vi "SVFA Power Spectral Density Subset (N Ch).vi"(0 "scaled signals [EU]":waveform(dbl)[](array[waveform]), 2 "window":T7=1 items=["None"=0, "Hanning"=1, "Hamming"=2, "Blackman-Harris"=3, "Exact Blackman"=4, "Blackman"=5, "Flat Top"=6, "4 Term B-Harris "=7, "7 Term B-Harris"=8, "Low Sidelobe"=9, "Force"=64, "Exponential"=65, "Blackman Nuttall"=11, "Triangle"=30, "Bartlett-Hanning"=31, "Bohman"=32, "Parzen"=33, "Welch"=34, "Kaiser"=60, "Dolph-Chebyshev"=61, "Gaussian"=62], 3 "frequency range":T9={"start frequency"=1000.0, "stop frequency"=2000.0} {"stop frequency" min=0.0 format="%.2f"; "start frequency" min=0.0 format="%.2f"}, 4 "dB On (T)":bool=TRUE, 5 "error in (no error)":errorcluster, 6 "desired units":enum16{"EU^2 / Hz", "EU / sqrt(Hz)"}(ring), 7 "averaging parameters":T8={"averaging mode"=enum."No averaging", "weighting mode"=enum."Exponential", "number of averages"=10, "linear mode"=enum."One shot"}, 9 "restart averaging (F)":bool) -> (11 "averaging done":bool, 13 "averages completed":dbl, 14 "power spectral densities [EU^2 rms / Hz]":cluster{"f0":dbl, "df":dbl, "magnitude":dbl[]}[](array[cluster]) {"magnitude" format="%.2p"; "df" format="%.2p"; "f0" format="%.2p"}, 15 "unit labels":string[](array[string]), 18 "spectrum info":T1[](array[typedef]) {"x-axis units" items=["Time (s)"=0, "Frequency-CB (Hz)"=1, "Frequency-CPB (Hz)"=1248, "Frequency-Arbitrary (Hz)"=2357, "Quefrency (s)"=2, "Revolutions (rev)"=3, "Order"=4, "Speed (RPM)"=11, "Speed (rad/s)"=21, "Index"=65535]; "weighting filter" items=["Linear", "A-weighting", "B-weighting", "C-weighting", "ITU-R 468-4", "Dolby", "CCITT", "C-message", "Wb", "Wc", "Wd", "We", "Wf", "Wh", "Wj", "Wk", "Wm", "AES17 20 kHz lowpass", "AES17 40 kHz lowpass", "AES17 20 kHz highpass", "AES17 40 kHz highpass"]; "dB reference [EU]" format="%.2f"; "engineering units" items=["custom..."=0, "V"=1, "A"=21, "C"=30, "pC"=31, "s"=32, "-"=29, "Pa"=2, "N"=20, "g"=3, "m/s^2"=4, "m/s"=5, "m"=6, "mm/s"=12, "mm"=13, "micron/s"=14, "micron"=15, "in/s^2"=7, "in/s"=8, "in"=9, "mil/s"=10, "mil"=11, "rad/s^2"=16, "rad/s"=17, "rad"=18, "deg/s^2"=26, "deg/s"=27, "deg"=28, "RPM"=22, "cycle/s^2"=23, "Hz"=24, "cycle"=25, "strain"=19]; "spectral info"."window" items=["None "=0, "Hanning"=1, "Hamming"=2, "Blackman-Harris"=3, "Exact Blackman"=4, "Blackman"=5, "Flat Top"=6, "4 Term B-Harris "=7, "7 Term B-Harris"=8, "Low Sidelobe"=9, "Force - Exponential"=10, "Gaussian"=62]}, 19 "error out":errorcluster)   [LabVIEW 2017]
doc: "Computes a subset of the power spectral density of <B>scaled signal [EU]</B>. The subset is defined by <B>frequency range</B>. Each block of data corresponds to a single FFT block and has to be passed individually to this VI. Wire data to the <B>scaled signal [EU]</B> input to determine the polymorphic instance to use or manually select the instance."
uses:
  <vilib>/addons/_NISVFA/_Shared subVIs/Controls/svc_Window.ctl
  <vilib>/addons/_NISVFA/_Shared subVIs/Controls/svc_Spectrum Info.ctl
  <vilib>/addons/_NISVFA/_Shared subVIs/Controls/svc_X-Axis Units.ctl
  <vilib>/addons/_NISVFA/_Shared subVIs/Controls/svc_Spectrum Type.ctl
  <vilib>/addons/_NISVFA/_Shared subVIs/Controls/svc_Engineering Units Text Ring.ctl
  <vilib>/addons/_NISVFA/_Shared subVIs/Controls/svc_Weighting Filter Text Ring.ctl
  <vilib>/addons/_NISVFA/_Shared subVIs/Controls/svc_Complimentary Spectrum Units.ctl
  <vilib>/addons/_NISVFA/_Shared subVIs/Windowing/svfa_Scaled Time Domain Window (1 Ch).vi
  <vilib>/addons/_NISVFA/_Shared subVIs/Spectrum Info/svfa_Build Spectrum Info.vi
  <vilib>/addons/_NISVFA/_Shared subVIs/Spectrum Averaging/svfa_Reset Averaging State Info.vi
  <vilib>/addons/_NISVFA/_Shared subVIs/Spectrum Averaging/svfa_Average Array with Avg Checks (complex) No State.vi
  <vilib>/addons/_NISVFA/_Shared subVIs/Common/svc_Complex to Mag2 Array.vi
  <vilib>/addons/_NISVFA/_Shared subVIs/Spectrum Averaging/svfa_Average Array with Avg Checks (real) No State.vi
  <vilib>/addons/_NISVFA/_Shared subVIs/Windowing/svfa_Scaled Time Domain Window (Array).vi
  <vilib>/addons/_NISVFA/_Shared subVIs/Common/svc_Get SV Channel Info.vi
  <vilib>/addons/_NISVFA/_Shared subVIs/Common/svc_Spectrum Units.vi
  <vilib>/addons/_NISVFA/_Shared subVIs/Spectrum Averaging/svfa_Average Array (complex) No State.vi
  <vilib>/addons/_NISVFA/_Shared subVIs/Spectrum Averaging/svfa_Average Array (real) No State.vi
  <vilib>/Analysis/4window.llb/Force Window.vi
  <vilib>/Analysis/4window.llb/Force Window (DBL).vi
  <vilib>/Analysis/4window.llb/Exponential Window.vi
  <vilib>/Analysis/4window.llb/Exponential Window (DBL).vi
  <vilib>/addons/_NISVFA/_Shared subVIs/Spectrum Averaging/svfa_No Average Array (complex).vi
  <vilib>/addons/_NISVFA/_Shared subVIs/Spectrum Averaging/svfa_Average Array (complex).vi
  <vilib>/addons/_NISVFA/_Shared subVIs/Spectrum Averaging/svfa_No Average Array (real).vi
  <vilib>/addons/_NISVFA/_Shared subVIs/Spectrum Averaging/svfa_Average Array (real).vi
  <vilib>/addons/_NISVFA/_Shared subVIs/Spectrum Averaging/svfa_Peak Hold Array.vi
  <vilib>/addons/_NISVFA/_Spectrum Processing/SVFA Unit Conversion (N Ch).vi
  <vilib>/addons/_NISVFA/_Shared subVIs/Common/svc_Get Weighting Enum and Labels.vi
  <vilib>/addons/_NISVFA/_Shared subVIs/Common/svc_Unit Label Lexical Class.vi
  <vilib>/addons/_NISVFA/_Shared subVIs/Common/svc_Engineering Units to Unit Label.vi
  <vilib>/addons/_NISVFA/_Shared subVIs/Common/svc_Format Value (DBL).vi
  <vilib>/addons/_NISVFA/_Shared subVIs/Common/svc_Channel Info to Spectrum Info.vi
  <vilib>/addons/_NISVFA/_Shared subVIs/Common/svc_Unit Label to Engineering Units.vi
  <vilib>/Utility/error.llb/Error Cluster From Error Code.vi
  <vilib>/Analysis/0measdsp.llb/Scaled Time Domain Window.vi
  <vilib>/Analysis/0measdsp.llb/Scaled Time Domain Window (DBL).vi
  <vilib>/addons/_NISVFA/_Spectrum Processing/subVIs/svfa_Spectrum Info Window to windowTd Type Def.vi
  <vilib>/addons/_NISVFA/_Shared subVIs/Common/svc_Window Parameters.vi
  <vilib>/addons/_NISVFA/_Shared subVIs/Common/svc_Get Window Info.vi
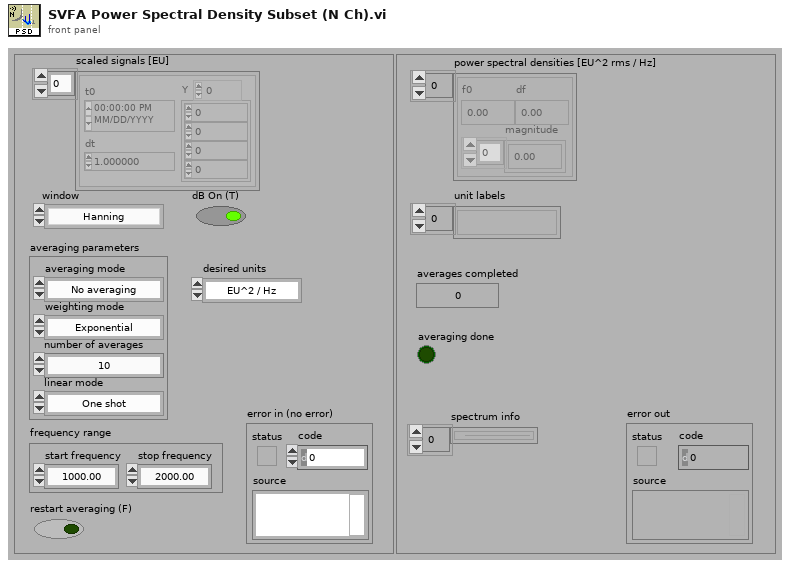
[diagram p1: front panel]
types:
  T1 = typedef "svc_Spectrum Info.ctl" = cluster{"channel name":string, "description":string, "x-axis units":T2, "spectral info":cluster{"spectrum type":T3, "linear/dB":enum16{"linear", "dB"}, "window":u16, "window size":i32, "FFT size":i32}, "engineering units":T4, "custom label":string, "dB reference [EU]":dbl, "peak units":enum16{"rms", "peak", "peak-peak"}, "weighting filter":T5, "spectral density?":bool, "unit label":string, "spectrum skewed?":bool, "complimentary spectrum units":T6}
  T2 = typedef "svc_X-Axis Units.ctl" = u16
  T3 = typedef "svc_Spectrum Type.ctl" = enum16{"FFT Spectrum [complex]", "Amplitude [Magnitude]", "Power [Magnitude^2]", "Cross Spectrum [complex]", "Frequency Response [Complex]"}
  T4 = typedef "svc_Engineering Units Text Ring.ctl" = u16
  T5 = typedef "svc_Weighting Filter Text Ring.ctl" = u16
  T6 = typedef "svc_Complimentary Spectrum Units.ctl" = enum16{"none", "radians", "degrees", "cycles", "imaginary"}
  T7 = typedef "svc_Window.ctl" = u32
  T8 = cluster{"averaging mode":enum16{"No averaging", "Vector averaging", "RMS averaging", "Peak hold"}, "weighting mode":enum16{"Linear", "Exponential"}, "number of averages":u32, "linear mode":enum16{"One shot", "Auto restart"}}
  T9 = cluster{"start frequency":dbl, "stop frequency":dbl}
  T10 = cluster{"linear/dB":enum16{"no change", "linear", "dB"}, "dB reference (0: no change)":dbl, "power/magnitude":enum16{"no change", "power", "magnitude"}, "view":enum16{"no change", "rms", "peak", "peak-peak"}}
  T11 = enum16{"no change", "spectrum", "spectral density"}
  T12 = enum16{"Restart processing", "Continue processing", "Skip processing"}
  T13 = cluster{"complex FFT":cdb[], "real FFT":dbl[], "f0":dbl, "df":dbl, "averages completed":dbl, "averaging parameters":cluster{"averaging mode":enum16{"No averaging", "Vector averaging", "RMS averaging", "Peak hold"}, "weighting mode":enum16{"Linear", "Exponential"}, "number of averages":u32, "linear mode":enum16{"One shot", "Auto restart"}}}[]
  T14 = enum16{"No averaging", "Vector averaging", "RMS averaging", "Peak hold"}
  T15 = cluster{"complex FFT":cdb[], "real FFT":dbl[], "f0":dbl, "df":dbl, "averages completed":dbl, "averaging parameters":cluster{"averaging mode":enum16{"No averaging", "Vector averaging", "RMS averaging", "Peak hold"}, "weighting mode":enum16{"Linear", "Exponential"}, "number of averages":u32, "linear mode":enum16{"One shot", "Auto restart"}}}
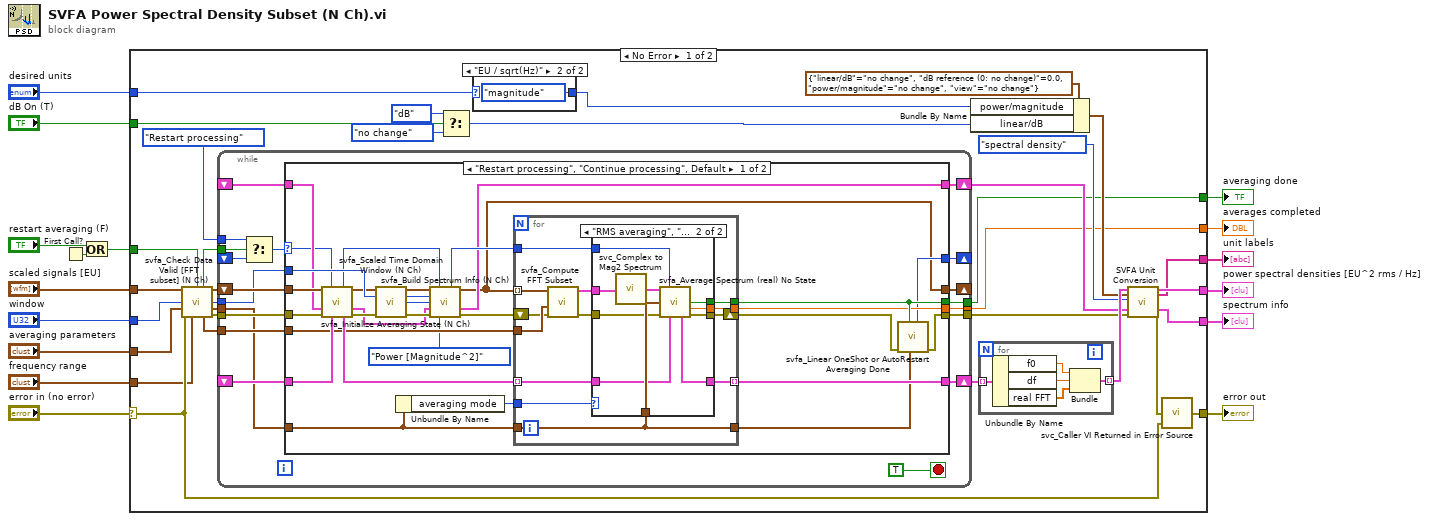
[diagram p0: block diagram]
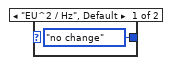
[diagram p2: hidden frame]
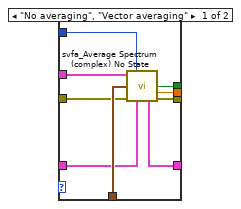
[diagram p3: hidden frame]
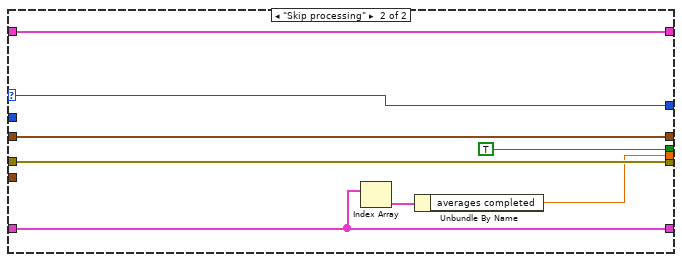
[diagram p4: hidden frame]
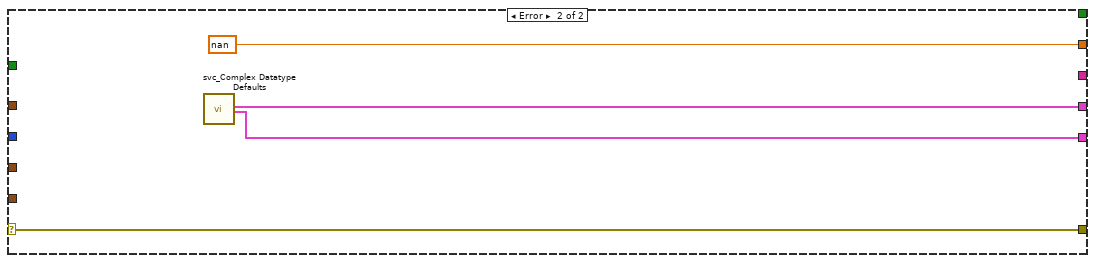
[diagram p5: hidden frame]
diagram:
  n1 = First Call?() -> (First Call?: T/F=w4:bool)
  n2 = Or(x="restart averaging (F)", y=w4) -> (x .or. y?=w3:bool)
  n3 = case shown="No Error" "error in (no error)" {
    selector: "error in (no error)" -> [w40 w149]
    tunnel: w3 -> [w47 _]
    tunnel: [w18 nan ("Averaged So-far")] -> w16
    tunnel: [w17 _] -> w15
    tunnel: [w45 w147] -> w10
    tunnel: [w42 w149] -> w14
    tunnel: "averaging parameters" -> [w46 _]
    tunnel: "frequency range" -> [w32 _]
    tunnel: "scaled signals [EU]" -> [w49 _]
    tunnel: "window" -> [w48 _]
    tunnel: [w44 _] -> w7
    tunnel: "dB On (T)" -> [w24 _]
    tunnel: [w41 w146] -> w5
    tunnel: "desired units" -> [w23 _]
    frame No Error {
      n4 = call <vilib>:"svfa_Check Data Valid [FFT subset] (N Ch).vi"("scaled signals"=w49, "restart averaging (F)"=w47, "window"=w48, "averaging parameters"=w46, "error in (no error)"=w40, "frequency range in"=w32) -> ("restart averaging"=w31:bool, "dup scaled signals"=w37:waveform(dbl)[], "window"=w36:u16, "dup averaging parameters"=w35:T8, "frequency range out"=w33:T9, "error out"=w34:errorcluster)  [unwired: 4 in]
      n5 = while {
        shift-left: _ -> [w65]
        shift-right: [w66] -> w39
        tunnel: [w72] -> w18
        tunnel: [w73] -> w17
        tunnel: [w74] -> w20
        tunnel: w34 -> [w70]
        tunnel: w33 -> [w75]
        shift-right: [w68] -> w19
        shift-left: _ -> [w67]
        shift-right: [w64] -> _
        shift-left: _ -> [w63]
        tunnel: w36 -> [w61]
        tunnel: w35 -> [w60]
        tunnel: T12."Restart processing" ("processing control in") -> [w59]
        tunnel: w31 -> [w58]
        shift-right: [w57] -> _
        shift-left: w37 -> [w71]
        stop <- TRUE stop-if-true
        n6 = Select(t=w59, s=w58, f=w63) -> (s? t:f=w62:T12)
        n7 = case shown="\"Restart processing\", \"Continue processing\", Default" w62 {
          selector: w62 -> [w79 w143]
          tunnel: w75 -> [w88 _]
          tunnel: w60 -> [w98 _]
          tunnel: [w78 w139] -> w68
          tunnel: [w104 w141] -> w66
          tunnel: [w97 w144] -> w74
          tunnel: [w102 TRUE ("averaging done?")] -> w73
          tunnel: [w101 w142] -> w72
          tunnel: w71 -> [w95 w138]
          tunnel: w70 -> [w94 w144]
          tunnel: w67 -> [w89 w139]
          tunnel: w65 -> [w93 w141]
          tunnel: [w99 w143] -> w64
          tunnel: w61 -> [w100 _]
          tunnel: [w76 w138] -> w57
          frame "Restart processing", "Continue processing", Default {
            n8 = call <vilib>:"svfa_Initialize Averaging State (N Ch).vi"("Windowed Waveform(s)"=w95, "processing control in"=w79, "spectra info in"=w89, "error in (no error)"=w94, "state info"=w93) -> ("processing control out"=w77:T12, "Windowed Waveform(s)"=w91:waveform(dbl)[], "spectra info out"=w80:T1[], "state info"=w92:T13, "error out"=w90:errorcluster)  [unwired: 6 in]
            n9 = call <vilib>:"svfa_Scaled Time Domain Window (N Ch).vi"("Scaled signal(s)"=w91, "window"=w100, "error in (no error)"=w90) -> ("Windowed Waveform(s)"=w87:waveform(dbl)[], "window"=w84:T7, "window length"=w83:i32, "error out"=w82:errorcluster)  [unwired: 8 in, 1 out]
            n10 = Unbundle By Name(w98) -> ("averaging mode"=w105:T14)
            n11 = call <vilib>:"svfa_Build Spectrum Info (N Ch).vi"("scaled signal(s)"=w87, "processing control in"=w77, "window"=w84, "window size"=w83, "spectra info in"=w80, "error in (no error)"=w82, "spectrum type"=svc_Spectrum_Type."Power [Magnitude^2]" ("spectrum type 2")) -> ("dup processing control"=w86:T12, "dup scaled signals"=w76:waveform(dbl)[], "spectra info out"=w78:T1[], "error out"=w81:errorcluster)  [unwired: 5 in]
            n12 = for {
              tunnel: w105 -> [w118]
              tunnel: [w111] -> w104 mode=indexing
              tunnel: [w116] -> w102
              tunnel: [w115] -> w101
              tunnel: w86 -> [w114]
              tunnel: w98 -> [w112]
              tunnel: w92 -> [w113] mode=indexing
              tunnel: [w112] -> w96
              shift-right: [w117] -> w103
              shift-left: w81 -> [w108]
              tunnel: w88 -> [w109]
              tunnel: w76 -> [w110] mode=indexing
              n13 = call <vilib>:"svfa_Compute FFT Subset.vi"("error in (no error)"=w108, "frequency range"=w109, "windowed signal"=w110) -> ("error out"=w107:errorcluster, "FFT spectrum [Vrms]"=w106:cluster{"f0":dbl, "df":dbl, "spectrum":cdb[]})  [unwired: 7 in]
              n14 = case shown="\"RMS averaging\", \"Peak hold\"" w118 {
                tunnel: w112 -> [w127 w133]
                tunnel: [w119 w130] -> w111
                tunnel: [w126 w136] -> w117
                tunnel: [w125 w137] -> w116
                tunnel: w107 -> [w120 w129]
                tunnel: w114 -> [w123 w132]
                tunnel: [w124 w135] -> w115
                tunnel: w113 -> [w122 w131]
                tunnel: w106 -> [w121 w128]
                frame "No averaging", "Vector averaging" {
                  n15 = call <vilib>:"svfa_Average Spectrum (complex) No State.vi"("spectrum"=w121, "processing control"=w123, "averaging parameters"=w127, "error in (no error)"=w120, "averaging state info in"=w122) -> ("averaging done"=w125:bool, "averages completed"=w124:dbl, "averaging state info out"=w119:T15, "error out"=w126:errorcluster)  [unwired: 5 in, 2 out]
                }
                frame "RMS averaging", "Peak hold" {
                  n16 = call <vilib>:"svc_Complex to Mag2 Spectrum.vi"("complex spectrum"=w128) -> ("power spectrum"=w134:cluster{"f0":dbl, "df":dbl, "spectrum":dbl[]})  [unwired: 4 in]
                  n17 = call <vilib>:"svfa_Average Spectrum (real) No State.vi"("spectrum"=w134, "processing control"=w132, "averaging parameters"=w133, "error in (no error)"=w129, "averaging state info in"=w131) -> ("averaging done"=w137:bool, "averages completed"=w135:dbl, "averaging state info out"=w130:T15, "error out"=w136:errorcluster)  [unwired: 5 in, 2 out]
                }
              }
            }
            n18 = call <vilib>:"svfa_Linear OneShot or AutoRestart Averaging Done.vi"("averaging parameters"=w96, "averaging done"=w102, "error in (no error)"=w103) -> ("error out"=w97:errorcluster, "processing control"=w99:T12)  [unwired: 7 in]
          }
          frame "Skip processing" {
            n19 = Index Array(array=w141) -> (element=w140:T15)  [unwired: 1 in]
            n20 = Unbundle By Name(w140) -> ("averages completed"=w142:dbl)
          }
        }
      }
      n21 = Select(t=enum16{"no change", "linear", "dB"}."dB" ("linear/dB"), s=w24, f=enum16{"no change", "linear", "dB"}."no change" ("linear/dB")) -> (s? t:f=w27:enum16{"no change", "linear", "dB"})
      n22 = case shown="\"EU / sqrt(Hz)\"" w23 {
        tunnel: [enum16{"no change", "power", "magnitude"}."no change" ("power/magnitude") enum16{"no change", "power", "magnitude"}."magnitude" ("power/magnitude")] -> w29
        frame "EU^2 / Hz", Default {
        }
        frame "EU / sqrt(Hz)" {
        }
      }
      n23 = Bundle By Name(cluster=T10 {"linear/dB"=enum."no change", "dB reference (0: no change)"=0.0, "power/magnitude"=enum."no change", "view"=enum."no change"} ("desired scaling"), "power/magnitude"=w29, "linear/dB"=w27) -> (w22:T10)
      n24 = for {
        tunnel: w39 -> [w53] mode=indexing
        tunnel: [w52] -> w30 mode=indexing
        n25 = Unbundle By Name(w53) -> ("f0"=w54:dbl, "df"=w55:dbl, "real FFT"=w56:dbl[])
        n26 = Bundle("f0"=w54, "df"=w55, "real FFT"=w56) -> (w52:cluster{"f0":dbl, "df":dbl, "real FFT":dbl[]})  [unwired: 1 in]
      }
      n27 = call-poly <vilib>:"SVFA Unit Conversion.vi"("spectra"=w30, "desired scaling"=w22, "spectral density desired"=T11."spectral density", "spectrum info in"=w19, "error in (no error)"=w20) -> ("converted spectra"=w45:cluster{"x0":dbl, "dx":dbl, "magnitude":dbl[]}[], "unit labels"=w44:string[], "spectrum info out"=w41:T1[], "error out"=w43:errorcluster)  [unwired: 11 in]
      n28 = call <vilib>:"svc_Caller VI Returned in Error Source.vi"("warning input to caller"=w40, "error in (no error)"=w43) -> ("error out"=w42:errorcluster)  [unwired: 3 in]
    }
    frame Error {
      n29 = call <vilib>:"svc_Complex Datatype Defaults.vi"() -> ("empty array of spectra"=w147:cluster{"f0":dbl, "df":dbl, "magnitude":dbl[]}[], "empty array of spectrum info"=w146:T1[])  [unwired: 11 in, 7 out]
    }
  }
  "averages completed" <- w16
  "averaging done" <- w15
  "error out" <- w14
  "power spectral densities [EU^2 rms / Hz]" <- w10
  "unit labels" <- w7
  "spectrum info" <- w5
